vi "Preload Transient Configuration.vi"(9 "Value":variant, 10 "Name":string, 11 "TransientConfiguration in":refnum<class "TransientConfiguration.lvclass">) -> (3 "TransientConfiguration out":refnum<class "TransientConfiguration.lvclass">)   [LabVIEW 2019, in "TransientConfiguration.lvclass"]
uses:
  <vilib>/gpm_packages/@cs/Configuration/Source/TransientConfiguration/TransientConfiguration.lvclass
  <vilib>/gpm_packages/@cs/Configuration/Source/TransientConfiguration/TransientConfiguration.lvclass/TransientConfiguration.ctl
  <vilib>/Utility/Data Type/NI_Data Type.lvlib
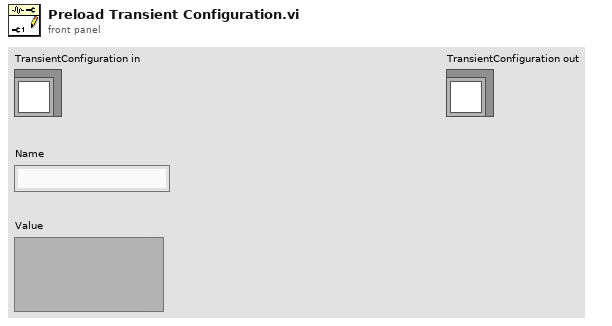
[diagram p1: front panel]
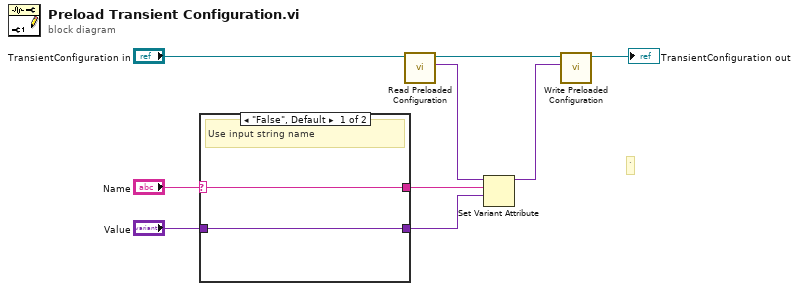
[diagram p0: block diagram]
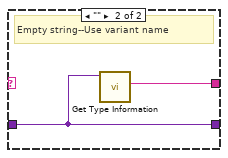
[diagram p2: hidden frame]
diagram:
  # "`"
  n1 = case shown="\"False\", Default" "Name" {
    selector: "Name" -> [w11 _]
    tunnel: "Value" -> [w10 w12]
    tunnel: [w10 w12] -> w2
    tunnel: [w11 w13] -> w1
    frame "False", Default {
      # "Use input string name"
    }
    frame "" {
      # "Empty string--Use variant name"
      n2 = call <vilib>:"Get Type Information.vi"("variant"=w12) -> ("name"=w13:string)  [unwired: 6 in, 4 out]
    }
  }
  n3 = call <vilib>:"Read Preloaded Configuration.vi"("TransientConfiguration in"="TransientConfiguration in") -> ("Pre-Loaded Configuration"=w6:variant, "TransientConfiguration out"=w8:refnum<class "TransientConfiguration.lvclass">)  [unwired: 9 in]
  n4 = Set Variant Attribute(Variant=w6, name=w1, value=w2) -> (Variant out=w5:variant)  [unwired: 1 in, 2 out]
  n5 = call <vilib>:"Write Preloaded Configuration.vi"("Pre-Loaded Configuration"=w5, "TransientConfiguration in"=w8) -> ("TransientConfiguration out"=→"TransientConfiguration out":refnum<class "TransientConfiguration.lvclass">)  [unwired: 9 in]
